vi "计算两条直线的交点（4点）.vi"(8 "Error In":errorcluster caption="错误输入", 10 "直线B":T1, 11 "直线A":T1) -> (0 "Error Out":errorcluster caption="错误输出", 3 "交点":T2)   [LabVIEW 2012, in "几何工具.lvlib"]
uses:
  <vilib>/Utility/miscctls.llb/LVPointDoubleTypeDef.ctl
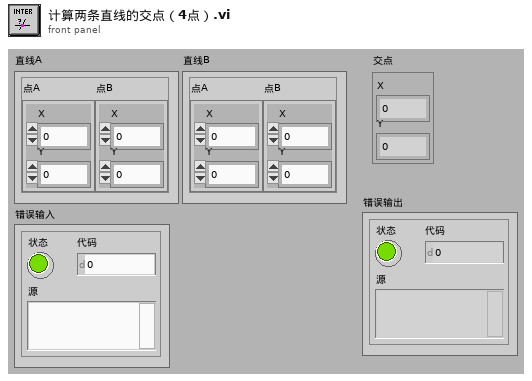
[diagram p1: front panel]
types:
  T1 = typedef "两点直线.ctl" = cluster{"点A":T2, "点B":T2}
  T2 = typedef "LVPointDoubleTypeDef.ctl" = cluster{"X":dbl, "Y":dbl}
  T3 = typedef "几何工具.lvlib/斜率与截距.ctl" = cluster{"斜率":dbl, "截距":dbl}
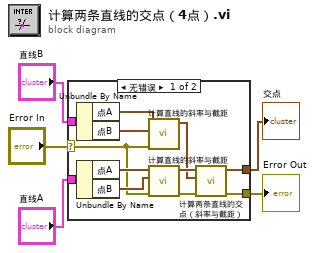
[diagram p0: block diagram]
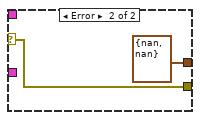
[diagram p2: hidden frame]
diagram:
  n1 = case shown="无错误" "Error In" {
    selector: "Error In" -> [w7 w19]
    tunnel: [w17 T2 {"X"=nan, "Y"=nan} ("交点")] -> w5
    tunnel: "直线A" -> [w16 _]
    tunnel: "直线B" -> [w13 _]
    tunnel: [w6 w19] -> w1
    frame No Error {
      n2 = Unbundle By Name(w13) -> ("点A"=w12:T2, "点B"=w11:T2)
      n3 = Unbundle By Name(w16) -> ("点A"=w15:T2, "点B"=w14:T2)
      n4 = call "计算直线的斜率与截距.vi"("Error In"=w7, "点B"=w11, "点A"=w12) -> ("斜率与截距"=w9:T3)  [unwired: 7 in, 1 out]
      n5 = call "计算直线的斜率与截距.vi"("Error In"=w7, "点B"=w14, "点A"=w15) -> ("Error Out"=w8:errorcluster, "斜率与截距"=w10:T3)  [unwired: 7 in]
      n6 = call "计算两条直线的交点（斜率与截距）.vi"("Error In"=w8, "直线B"=w9, "直线A"=w10) -> ("Error Out"=w6:errorcluster, "交点"=w17:T2)  [unwired: 7 in]
    }
    frame Error {
    }
  }
  "交点" <- w5
  "Error Out" <- w1
